vi "Export_spectrumFileName.vi"(0 "ITC503 Current Values":T2 {"ITC503 Gradient" format="%.2f"; "ITC503 Setpoint" min=-273.0 max=300000.0 step=0.0001 format="%.1f"; "ITC503 I" format="%_1f"; "ITC503 P" format="%_1f"; "ITC503 Temperature" min=0.0 max=1645.0 step=1e-05 format="%.2f"; "ITC503 Heater" min=0.0 max=100.0 step=0.01 scale=0.0..100.0}, 1 "iHR Current Values":T3={"iHR 550 Front Entrance"=0.0, "iHR550 Side Exit"=0.0, "iHR550 Wavelength"=897.9988, "iHR550 Exit Mirror"=2, "iHR550 Grating"="1", "Grating Index"=1} {"iHR550 Exit Mirror" items=["EntranceMirror", "ExitMirror", "Front", "Side"]}, 2 "Spectra Settings":T1={"Integration Time"=10.0, "Repetitions"=10, "Mapping Spectra"=TRUE} caption="Mapping Spectra Settings" {"Repetitions" min=1 max=100 step=1; "Integration Time" min=0.5 max=6000.0 step=1.0 format="%.1f"}, 3 "Drive Current Values":T4 {"Position"."Drive Z Position" min=-273.0 max=300000.0 step=0.0001 format="%.1f"; "Position"."Drive Y Position" min=-273.0 max=300000.0 step=0.0001 format="%.1f"; "Position"."Drive X Position" min=-273.0 max=300000.0 step=0.0001 format="%.1f"; "Voltages"."Drive Z Voltage" min=-273.0 max=300000.0 step=0.0001 format="%.1f"; "Voltages"."Drive Y Voltage" min=-273.0 max=300000.0 step=0.0001 format="%.1f"; "Voltages"."Drive X Voltage" min=-273.0 max=300000.0 step=0.0001 format="%.1f"}, 4 "CCD3500 Temperature":dbl caption="Temp. (°C)" min=10.0 max=160.0 step=0.1 format="%.1f") -> (5 "Filename":string)   [LabVIEW 2010]
uses:
  ESA-C/TypeDefs/ESA-C Current Values.ctl
  iHR550/TypeDefs/iHR Current Values.ctl
  ITC503/TypeDefs/ITC503 Current Values.ctl
  Mapping/TypeDefs/Mapping Spectra Params.ctl
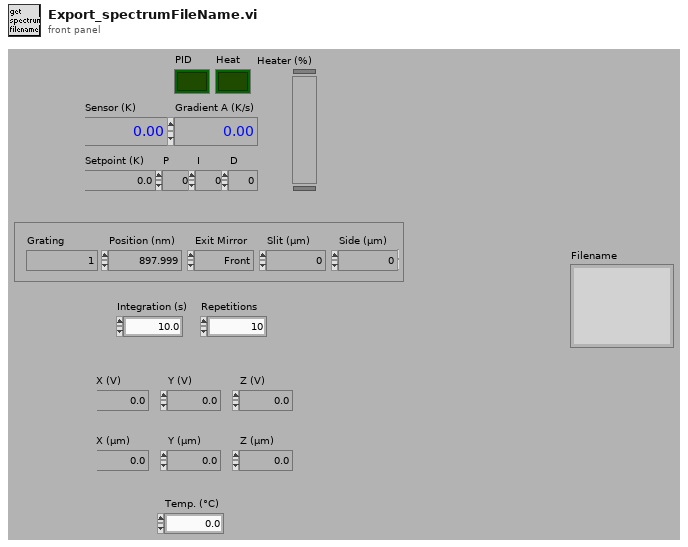
[diagram p1: front panel]
types:
  T1 = typedef "Mapping Spectra Params.ctl" = cluster{"Integration Time":dbl, "Repetitions":u16, "Mapping Spectra":bool}
  T2 = typedef "ITC503 Current Values.ctl" = cluster{"ITC503 Heater":dbl, "ITC503 Temperature":dbl, "ITC503 P":dbl, "ITC503 I":dbl, "ITC503 D":dbl, "ITC503 Setpoint":dbl, "ITC503 Gradient":dbl, "ITC503 Heater Auto":bool, "ITC503 PID Auto":bool}
  T3 = typedef "iHR Current Values.ctl" = cluster{"iHR 550 Front Entrance":dbl, "iHR550 Side Exit":dbl, "iHR550 Wavelength":dbl, "iHR550 Exit Mirror":i32, "iHR550 Grating":string, "Grating Index":i32}
  T4 = typedef "ESA-C Current Values.ctl" = cluster{"Voltages":cluster{"Drive X Voltage":dbl, "Drive Y Voltage":dbl, "Drive Z Voltage":dbl}, "Position":cluster{"Drive X Position":dbl, "Drive Y Position":dbl, "Drive Z Position":dbl}}
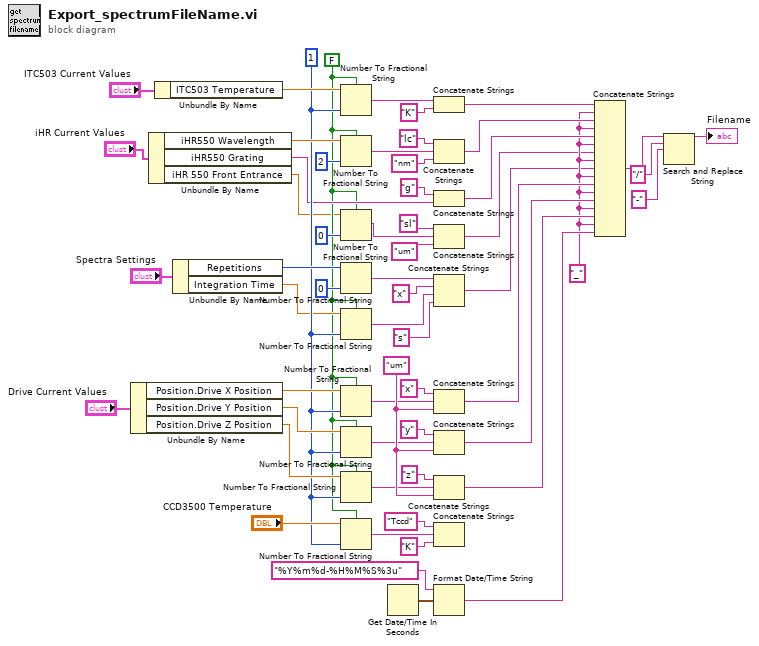
[diagram p0: block diagram]
diagram:
  w5 = "_" ("String")
  w32 = "um" ("String")
  w2 = FALSE ("Systemdezimalzeichen verwenden (T)")
  w46 = i16 1 ("Genauigkeit (6)")
  n1 = Unbundle By Name("Drive Current Values") -> ("Position.Drive X Position"=w52:dbl, "Position.Drive Y Position"=w51:dbl, "Position.Drive Z Position"=w50:dbl)
  n2 = Unbundle By Name("iHR Current Values") -> ("iHR550 Wavelength"=w49:dbl, "iHR550 Grating"=w24:string, "iHR 550 Front Entrance"=w1:dbl)
  n3 = Unbundle By Name("ITC503 Current Values") -> ("ITC503 Temperature"=w54:dbl)
  n4 = Unbundle By Name("Spectra Settings") -> ("Repetitions"=w53:u16, "Integration Time"=w38:dbl)
  n5 = Number To Fractional String(use system decimal point (T)=w2, number=w54, precision (6)=w46) -> (F-format string=w45:string)  [unwired: 1 in]
  n6 = Number To Fractional String(use system decimal point (T)=w2, number=w49, precision (6)=i16 2 ("Genauigkeit (6)")) -> (F-format string=w34:string)  [unwired: 1 in]
  n7 = Number To Fractional String(use system decimal point (T)=w2, number=w1, precision (6)=i16 0 ("Genauigkeit (6)")) -> (F-format string=w6:string)  [unwired: 1 in]
  n8 = Number To Fractional String(number=w53, precision (6)=i16 0 ("Genauigkeit (6)")) -> (F-format string=w41:string)  [unwired: 2 in]
  n9 = Number To Fractional String(use system decimal point (T)=w2, number=w38, precision (6)=w46) -> (F-format string=w40:string)  [unwired: 1 in]
  n10 = Number To Fractional String(use system decimal point (T)=w2, number=w52, precision (6)=w46) -> (F-format string=w31:string)  [unwired: 1 in]
  n11 = Number To Fractional String(use system decimal point (T)=w2, number=w51, precision (6)=w46) -> (F-format string=w30:string)  [unwired: 1 in]
  n12 = Number To Fractional String(use system decimal point (T)=w2, number=w50, precision (6)=w46) -> (F-format string=w29:string)  [unwired: 1 in]
  n13 = Number To Fractional String(use system decimal point (T)=w2, number="CCD3500 Temperature", precision (6)=w46) -> (F-format string=w37:string)  [unwired: 1 in]
  n14 = Get Date/Time In Seconds() -> (seconds since 1Jan1904=w12:timestamp)
  n15 = Concatenate Strings(w45, "K" ("String")) -> (w23:string)
  n16 = Concatenate Strings("lc" ("String"), w34, "nm" ("String")) -> (w22:string)
  n17 = Concatenate Strings("g" ("String"), w24) -> (w21:string)
  n18 = Concatenate Strings("sl" ("String"), w6, "um" ("String")) -> (w4:string)
  n19 = Concatenate Strings(w41, "x" ("String"), w40, "s" ("String")) -> (w3:string)
  n20 = Concatenate Strings("x" ("String"), w31, w32) -> (w20:string)
  n21 = Concatenate Strings("y" ("String"), w30, w32) -> (w19:string)
  n22 = Concatenate Strings("z" ("String"), w29, w32) -> (w18:string)
  n23 = Concatenate Strings("Tccd" ("String"), w37, "K" ("String")) -> ()  [unwired: 1 out]
  n24 = Format Date/Time String(time format string (%c)="%Y%m%d-%H%M%S%3u", seconds (now)=w12) -> (date/time string=w11:string)  [unwired: 1 in]
  n25 = Concatenate Strings(w23, w5, w22, w5, w21, w5, w4, w5, w3, w5, w20, w5, w19, w5, w18, w5, w11) -> (w16:string)
  n26 = Search and Replace String(input string=w16, search string="/" ("Such-String"), replace string="-" ("replace string (\"\")")) -> (result string=→"Filename":string)  [unwired: 5 in, 3 out]
